vi "List Topic Subscriptions.vi"(8 "error in (no error)":errorcluster, 11 "Topic in":refnum<class "Topic.lvclass">) -> (0 "error out":errorcluster, 2 "Subscriptions":refnum<class "Subscription.lvclass">[](array[class]), 3 "Topic out":refnum<class "Topic.lvclass">)   [LabVIEW 2015, in "NI_AWS_SNS.lvlib" / "Topic.lvclass"]
doc: "Returns a list of the subscriptions to a specific topic.\n\nThis action is throttled at 30 transactions per second (TPS)."
uses:
  Topic.lvclass
  Subscription/Subscription.lvclass
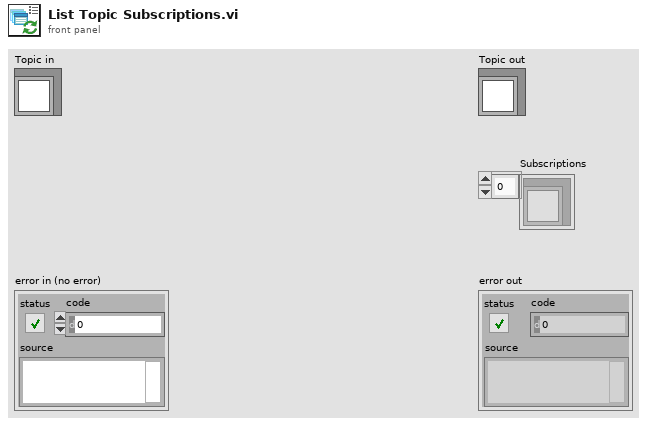
[diagram p1: front panel]
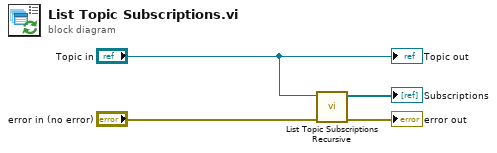
[diagram p0: block diagram]
diagram:
  n1 = call "List Topic Subscriptions Recursive.vi"("error in (no error)"="error in (no error)", "Topic"="Topic in") -> ("error out"=→"error out":errorcluster, "Topic Subscriptions"=→"Subscriptions":refnum<class "Subscription.lvclass">[])  [unwired: 8 in]
  "Topic out" <- "Topic in"
